vi "Create Value Set Blocking Callback.vi"(8 "error in (no error)":errorcluster, 10 "Scope":refnum<class "Future.lvclass">) -> (0 "error out":errorcluster, 2 "Synchronous Callback":refnum<class "Blocking Callback.lvclass">)   [LabVIEW 2017, in "Promise Future.lvlib" / "Future.lvclass"]
uses:
  Future.lvclass
  Callback/Blocking Callback.lvclass
  E:/Promise/Promise Future/Callback/Callback.lvclass
  Callback/Callback.lvclass/Callback.ctl
  Callback/Write Callback.vi
  Callback/Write Scope.vi
  Value Set Callback.vi
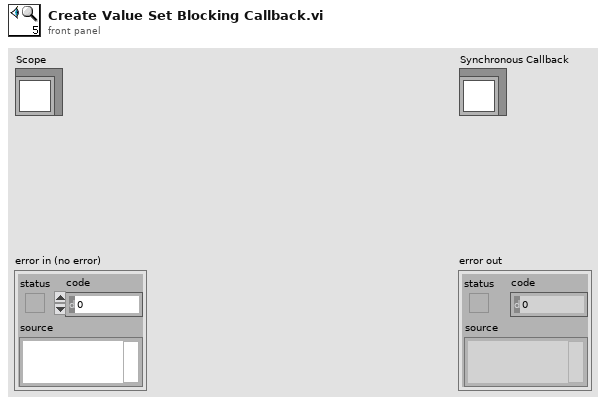
[diagram p1: front panel]
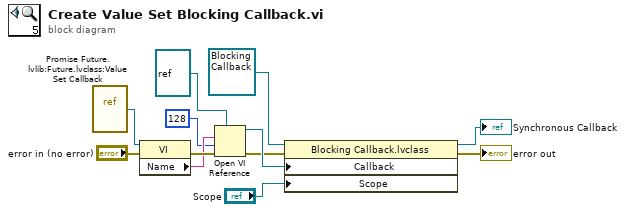
[diagram p0: block diagram]
diagram:
  n1 = vi-ref "Promise Future.lvlib:Future.lvclass:Value Set Callback.vi"() -> (w9:refnum<vi>)
  n2 = property class="VI"(reference=w9, error in="error in (no error)") -> (error out=w11:errorcluster, "Name"=w10:string)  [unwired: 1 out]
  n3 = Open VI Reference(type specifier VI Refnum (for type only)=refnum<vi> refnum, vi path=w10, options=128, error in (no error)=w11) -> (vi reference=w5:refnum<vi>, error out=w2:errorcluster)  [unwired: 2 in]
  n4 = property class="Blocking Callback.lvclass"(reference=refnum<class "Blocking Callback.lvclass"> refnum ("Synchronous Callback"), error in=w2, "Callback"=w5, "Scope"="Scope") -> (reference out=→"Synchronous Callback":refnum<class "Blocking Callback.lvclass">, error out=→"error out":errorcluster)
